vi "LVClass_SlopesPostProcessList AddProcessorTab.vi"(0 "SlopesPostProcessorList in":refnum<class "SlopesPostProcessorList.lvclass">, 5 "Processor List":T1[](array[typedef]), 11 "error in (no error)":errorcluster) -> (4 "SlopesPostProcessorList out":refnum<class "SlopesPostProcessorList.lvclass">, 15 "error out":errorcluster)   [LabVIEW 2020, in "SlopesPostProcessorList.lvclass"]
uses:
  SlopesPostProcessorList.lvclass
  SlopesPostProcessorList - ONE.ctl
  SlopesPostProcessorList - Filter.ctl
  SlopesPostProcessorList - Add lens.ctl
  SlopesPostProcessorList - Double passage.ctl
  HasoSlopes.lvclass
  SlopesPostProcessorList.lvclass/SlopesPostProcessorList.ctl
  Pupil.lvclass
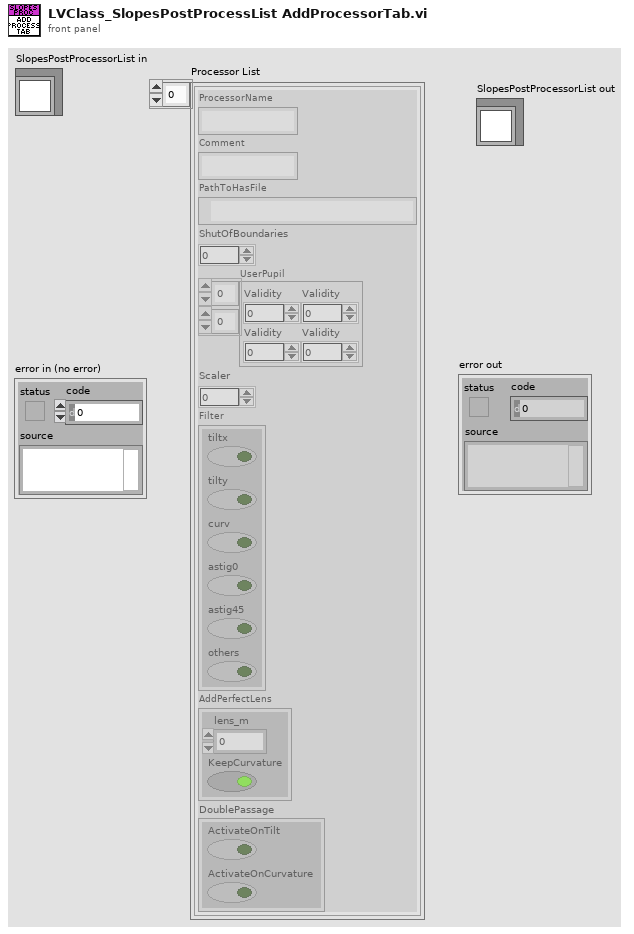
[diagram p1: front panel]
types:
  T1 = typedef "SlopesPostProcessorList - ONE.ctl" = cluster{"ProcessorName":string, "Comment":string, "PathToHasFile":path, "ShutOfBoundaries":u16, "UserPupil":i8[][], "Scaler":sgl, "Filter":T2, "AddPerfectLens":T3, "DoublePassage":T4}
  T2 = typedef "SlopesPostProcessorList - Filter.ctl" = cluster{"tiltx":bool, "tilty":bool, "curv":bool, "astig0":bool, "astig45":bool, "others":bool}
  T3 = typedef "SlopesPostProcessorList - Add lens.ctl" = cluster{"lens_m":sgl, "KeepCurvature":bool}
  T4 = typedef "SlopesPostProcessorList - Double passage.ctl" = cluster{"ActivateOnTilt":bool, "ActivateOnCurvature":bool}
  T5 = typedef "General dimensions definition.ctl" = cluster{"Size":T6, "Step":T7}
  T6 = typedef "Point2D.ctl" = cluster{"X":u32, "Y":u32}
  T7 = typedef "Point2Df.ctl" = cluster{"X":sgl, "Y":sgl}
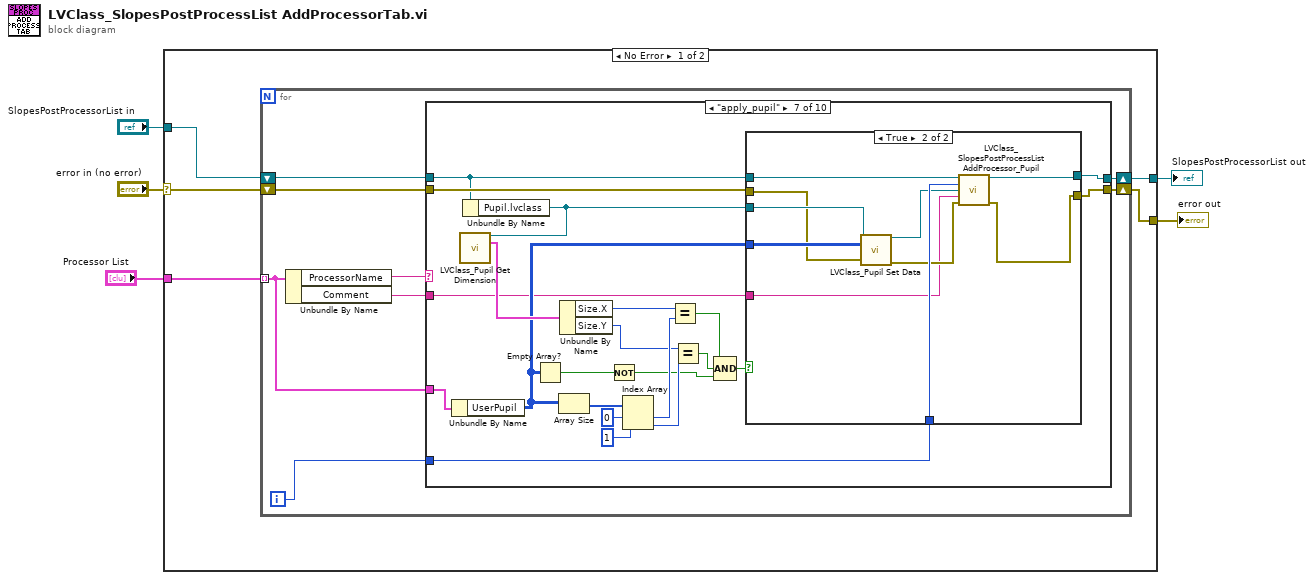
[diagram p0: block diagram]
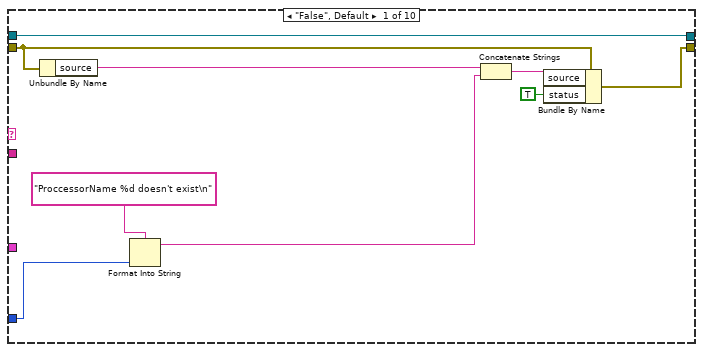
[diagram p2: hidden frame]
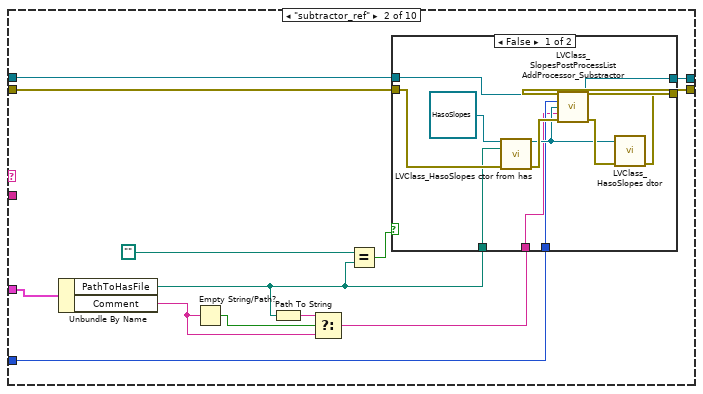
[diagram p3: hidden frame]
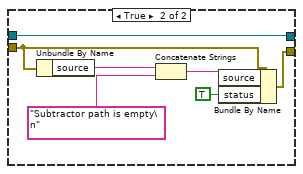
[diagram p4: hidden frame]
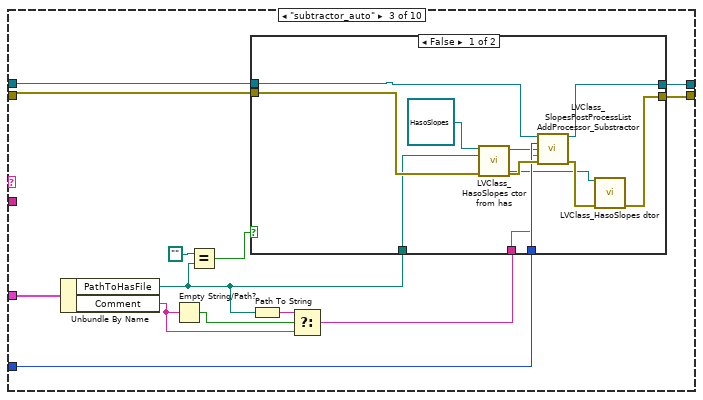
[diagram p5: hidden frame]
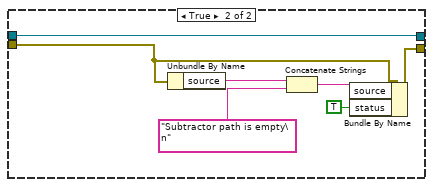
[diagram p6: hidden frame]
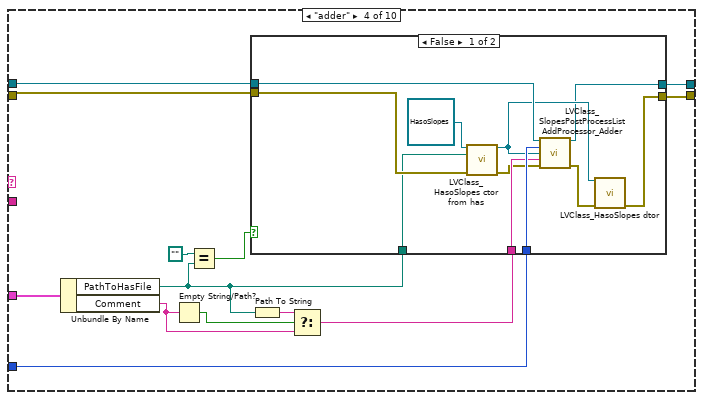
[diagram p7: hidden frame]
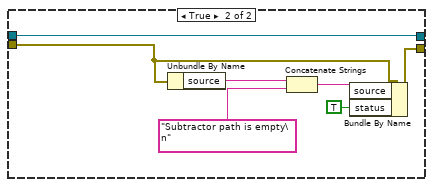
[diagram p8: hidden frame]
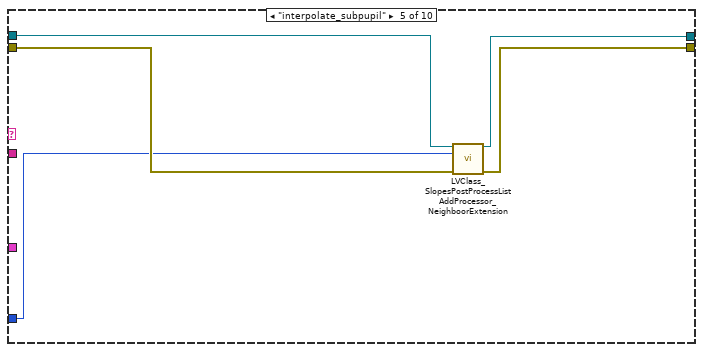
[diagram p9: hidden frame]
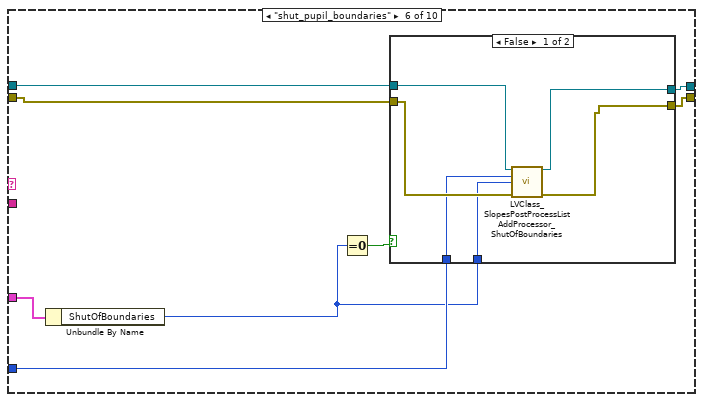
[diagram p10: hidden frame]
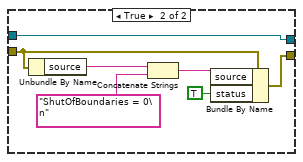
[diagram p11: hidden frame]
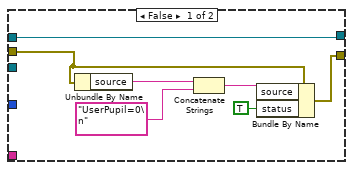
[diagram p12: hidden frame]
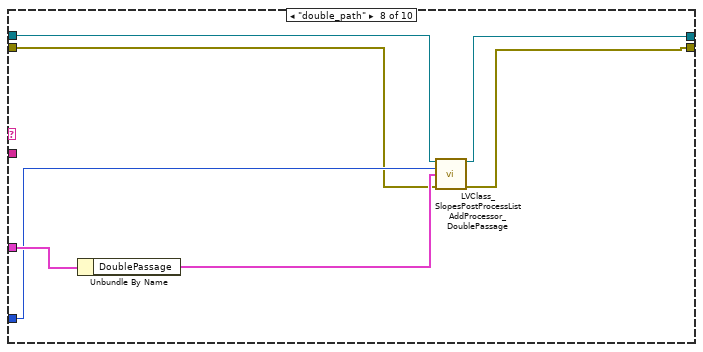
[diagram p13: hidden frame]
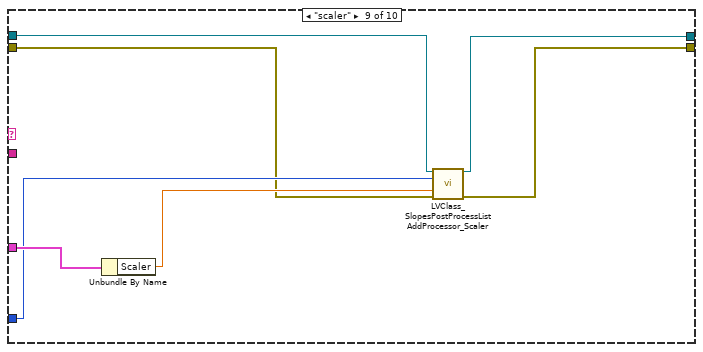
[diagram p14: hidden frame]
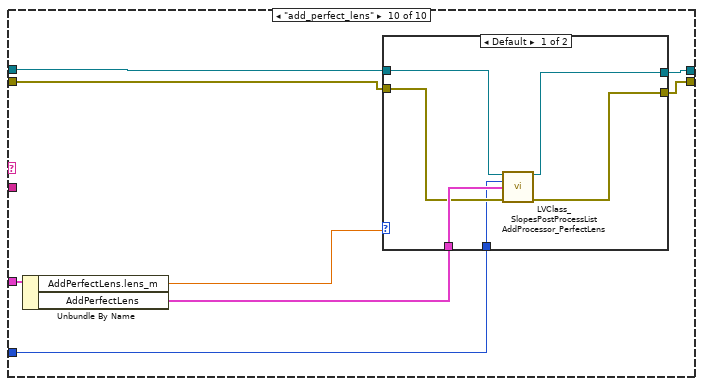
[diagram p15: hidden frame]
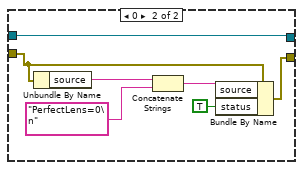
[diagram p16: hidden frame]
diagram:
  n1 = case shown="No Error" "error in (no error)" {
    selector: "error in (no error)" -> [w10 w221]
    tunnel: [w6 w221] -> w4
    tunnel: [w7 w222] -> w2
    tunnel: "SlopesPostProcessorList in" -> [w8 w222]
    tunnel: "Processor List" -> [w9 _]
    frame No Error {
      n2 = for {
        tunnel: w9 -> [w17] mode=indexing
        shift-right: [w15] -> w6
        shift-left: w10 -> [w16]
        shift-right: [w12] -> w7
        shift-left: w8 -> [w13]
        i -> [w14]
        n3 = Unbundle By Name(w17) -> ("ProcessorName"=w18:string, "Comment"=w11:string)
        n4 = case shown="\"apply_pupil\"" w18 {
          tunnel: w17 -> [_ w40 w71 w102 _ w133 w168 w192 w199 w207]
          tunnel: w16 -> [w27 w39 w68 w99 w123 w131 w167 w187 w194 w205]
          tunnel: [w26 w38 w67 w98 w122 w130 w166 w186 w193 w206] -> w15
          tunnel: w14 -> [w22 w33 w64 w95 w121 w127 w163 w190 w196 w200]
          tunnel: w13 -> [w19 w35 w66 w97 w125 w129 w162 w189 w198 w202]
          tunnel: [w19 w34 w65 w96 w124 w128 w164 w188 w197 w201] -> w12
          tunnel: w11 -> [_ _ _ _ _ _ w147 _ _ _]
          frame "False", Default {
            n5 = Unbundle By Name(w27) -> ("source"=w24:string)
            n6 = Format Into String(format string="ProccessorName %d doesn't exist\n" ("source"), w22) -> (resulting string=w21:string)  [unwired: 2 in, 1 out]
            n7 = Concatenate Strings(w24, w21) -> (w23:string)
            n8 = Bundle By Name(cluster=w27, "source"=w23, "status"=TRUE) -> (w26:errorcluster)
          }
          frame "subtractor_ref" {
            n9 = Unbundle By Name(w40) -> ("PathToHasFile"=w29:path, "Comment"=w30:string)
            n10 = Empty String/Path?(string/path=w30) -> (empty?=w31:bool)
            n11 = Path To String(path=w29) -> (string=w32:string)
            n12 = Select(t=w32, s=w31, f=w30) -> (s? t:f=w28:string)
            n13 = Equal?(x=path "", y=w29) -> (x = y?=w36:bool)
            n14 = case shown="False" w36 {
              tunnel: w39 -> [w47 w54]
              tunnel: [w46 w55] -> w38
              tunnel: w35 -> [w45 w52]
              tunnel: [w44 w52] -> w34
              tunnel: w33 -> [w43 _]
              tunnel: w29 -> [w42 _]
              tunnel: w28 -> [w41 _]
              frame False {
                n15 = call "LVClass_HasoSlopes ctor from has.vi"("HasoSlopes (const)"=refnum<class "HasoSlopes.lvclass"> refnum ("HasoSlopes in"), ".has path"=w42, "error in (no error)"=w47) -> ("HasoSlopes (new)"=w48:refnum<class "HasoSlopes.lvclass">, "error out"=w50:errorcluster)  [unwired: 11 in]
                n16 = call "LVClass_SlopesPostProcessList AddProcessor_Substractor.vi"("SlopesPostProcessorList in"=w45, "Position"=w43, "HasoSlopes.lvclass"=w48, "Comment"=w41, "error in (no error)"=w50) -> ("SlopesPostProcessorList out"=w44:refnum<class "SlopesPostProcessorList.lvclass">, "error out"=w49:errorcluster)  [unwired: 9 in]
                n17 = call "LVClass_HasoSlopes dtor.vi"("HasoSlopes in"=w48, "error in (no error)"=w49) -> ("error out"=w46:errorcluster)  [unwired: 12 in, 1 out]
              }
              frame True {
                n18 = Unbundle By Name(w54) -> ("source"=w57:string)
                n19 = Concatenate Strings(w57, "Subtractor path is empty\n" ("source")) -> (w56:string)
                n20 = Bundle By Name(cluster=w54, "source"=w56, "status"=TRUE) -> (w55:errorcluster)
              }
            }
          }
          frame "subtractor_auto" {
            n21 = Unbundle By Name(w71) -> ("PathToHasFile"=w63:path, "Comment"=w61:string)
            n22 = Empty String/Path?(string/path=w61) -> (empty?=w60:bool)
            n23 = Equal?(x=path "", y=w63) -> (x = y?=w69:bool)
            n24 = Path To String(path=w63) -> (string=w62:string)
            n25 = Select(t=w62, s=w60, f=w61) -> (s? t:f=w59:string)
            n26 = case shown="False" w69 {
              tunnel: w68 -> [w81 w85]
              tunnel: [w75 w84] -> w67
              tunnel: w63 -> [w73 _]
              tunnel: w66 -> [w79 w83]
              tunnel: [w78 w83] -> w65
              tunnel: w64 -> [w77 _]
              tunnel: w59 -> [w72 _]
              frame False {
                n27 = call "LVClass_HasoSlopes ctor from has.vi"("HasoSlopes (const)"=refnum<class "HasoSlopes.lvclass"> refnum ("HasoSlopes in"), ".has path"=w73, "error in (no error)"=w81) -> ("HasoSlopes (new)"=w74:refnum<class "HasoSlopes.lvclass">, "error out"=w80:errorcluster)  [unwired: 11 in]
                n28 = call "LVClass_SlopesPostProcessList AddProcessor_Substractor.vi"("SlopesPostProcessorList in"=w79, "Position"=w77, "HasoSlopes.lvclass"=w74, "Comment"=w72, "error in (no error)"=w80) -> ("SlopesPostProcessorList out"=w78:refnum<class "SlopesPostProcessorList.lvclass">, "error out"=w76:errorcluster)  [unwired: 9 in]
                n29 = call "LVClass_HasoSlopes dtor.vi"("HasoSlopes in"=w74, "error in (no error)"=w76) -> ("error out"=w75:errorcluster)  [unwired: 12 in, 1 out]
              }
              frame True {
                n30 = Unbundle By Name(w85) -> ("source"=w88:string)
                n31 = Concatenate Strings(w88, "Subtractor path is empty\n" ("source")) -> (w87:string)
                n32 = Bundle By Name(cluster=w85, "source"=w87, "status"=TRUE) -> (w84:errorcluster)
              }
            }
          }
          frame "adder" {
            n33 = Unbundle By Name(w102) -> ("PathToHasFile"=w94:path, "Comment"=w92:string)
            n34 = Empty String/Path?(string/path=w92) -> (empty?=w91:bool)
            n35 = Equal?(x=path "", y=w94) -> (x = y?=w100:bool)
            n36 = Path To String(path=w94) -> (string=w93:string)
            n37 = Select(t=w93, s=w91, f=w92) -> (s? t:f=w90:string)
            n38 = case shown="False" w100 {
              tunnel: w99 -> [w112 w116]
              tunnel: [w111 w115] -> w98
              tunnel: w94 -> [w110 _]
              tunnel: w97 -> [w109 w114]
              tunnel: [w104 w114] -> w96
              tunnel: w95 -> [w108 _]
              tunnel: w90 -> [w106 _]
              frame False {
                n39 = call "LVClass_HasoSlopes ctor from has.vi"("HasoSlopes (const)"=refnum<class "HasoSlopes.lvclass"> refnum ("HasoSlopes in"), ".has path"=w110, "error in (no error)"=w112) -> ("HasoSlopes (new)"=w107:refnum<class "HasoSlopes.lvclass">, "error out"=w105:errorcluster)  [unwired: 11 in]
                n40 = call "LVClass_SlopesPostProcessList AddProcessor_Adder.vi"("SlopesPostProcessorList in"=w109, "Position"=w108, "HasoSlopes.lvclass"=w107, "Comment"=w106, "error in (no error)"=w105) -> ("SlopesPostProcessorList out"=w104:refnum<class "SlopesPostProcessorList.lvclass">, "error out"=w103:errorcluster)  [unwired: 9 in]
                n41 = call "LVClass_HasoSlopes dtor.vi"("HasoSlopes in"=w107, "error in (no error)"=w103) -> ("error out"=w111:errorcluster)  [unwired: 12 in, 1 out]
              }
              frame True {
                n42 = Unbundle By Name(w116) -> ("source"=w119:string)
                n43 = Concatenate Strings(w119, "Subtractor path is empty\n" ("source")) -> (w118:string)
                n44 = Bundle By Name(cluster=w116, "source"=w118, "status"=TRUE) -> (w115:errorcluster)
              }
            }
          }
          frame "interpolate_subpupil" {
            n45 = call "LVClass_SlopesPostProcessList AddProcessor_NeighboorExtension.vi"("SlopesPostProcessorList in"=w125, "Position"=w121, "error in (no error)"=w123) -> ("SlopesPostProcessorList out"=w124:refnum<class "SlopesPostProcessorList.lvclass">, "error out"=w122:errorcluster)  [unwired: 11 in]
          }
          frame "shut_pupil_boundaries" {
            n46 = Unbundle By Name(w133) -> ("ShutOfBoundaries"=w126:u16)
            n47 = Equal To 0?(x=w126) -> (x = 0?=w132:bool)
            n48 = case shown="False" w132 {
              tunnel: w131 -> [w138 w141]
              tunnel: [w137 w142] -> w130
              tunnel: w129 -> [w139 w140]
              tunnel: [w136 w140] -> w128
              tunnel: w127 -> [w135 _]
              tunnel: w126 -> [w134 _]
              frame False {
                n49 = call "LVClass_SlopesPostProcessList AddProcessor_ShutOfBoundaries.vi"("SlopesPostProcessorList in"=w139, "Position"=w135, "ShutOfBoundaries"=w134, "error in (no error)"=w138) -> ("SlopesPostProcessorList out"=w136:refnum<class "SlopesPostProcessorList.lvclass">, "error out"=w137:errorcluster)  [unwired: 10 in]
              }
              frame True {
                n50 = Unbundle By Name(w141) -> ("source"=w145:string)
                n51 = Concatenate Strings(w145, "ShutOfBoundaries = 0\n" ("source")) -> (w144:string)
                n52 = Bundle By Name(cluster=w141, "source"=w144, "status"=TRUE) -> (w142:errorcluster)
              }
            }
          }
          frame "apply_pupil" {
            n53 = Unbundle By Name(w168) -> ("UserPupil"=w159:i8[][])
            n54 = Unbundle By Name(w162) -> ("Pupil.lvclass"=w161:refnum<class "Pupil.lvclass">)
            n55 = call "LVClass_Pupil Get Dimension.vi"("Pupil in"=w161) -> ("Dimension"=w160:T5)  [unwired: 12 in, 2 out]
            n56 = Empty Array?(array=w159) -> (empty?=w165:bool)
            n57 = Array Size(array=w159) -> (size(s)=w158:i32[])
            n58 = Unbundle By Name(w160) -> ("Size.X"=w155:u32, "Size.Y"=w153:u32)
            n59 = Not(x=w165) -> (.not. x?=w149:bool)
            n60 = Index Array(array=w158, index #1=0 ("index"), index #2=1 ("index")) -> (element #1=w154:i32, element #2=w152:i32)
            n61 = Equal?(x=w155, y=w154) -> (x = y?=w151:bool)
            n62 = Equal?(x=w153, y=w152) -> (x = y?=w150:bool)
            n63 = Compound Arithmetic op=AND(w151, w150, w149) -> (w148:bool)
            n64 = case shown="True" w148 {
              tunnel: w167 -> [w172 w178]
              tunnel: [w171 w177] -> w166
              tunnel: w162 -> [w169 w185]
              tunnel: [w169 w180] -> w164
              tunnel: w163 -> [_ w183]
              tunnel: w159 -> [_ w184]
              tunnel: w161 -> [_ w179]
              tunnel: w147 -> [_ w176]
              frame False {
                n65 = Unbundle By Name(w172) -> ("source"=w174:string)
                n66 = Concatenate Strings(w174, "UserPupil=0\n" ("source")) -> (w173:string)
                n67 = Bundle By Name(cluster=w172, "source"=w173, "status"=TRUE) -> (w171:errorcluster)
              }
              frame True {
                n68 = call "LVClass_Pupil Set Data.vi"("Pupil in"=w179, "Data"=w184, "error in (no error)"=w178) -> ("Pupil out"=w181:refnum<class "Pupil.lvclass">, "error out"=w182:errorcluster)  [unwired: 11 in]
                n69 = call "LVClass_SlopesPostProcessList AddProcessor_Pupil.vi"("SlopesPostProcessorList in"=w185, "Position"=w183, "Pupil.lvclass"=w181, "Comment"=w176, "error in (no error)"=w182) -> ("SlopesPostProcessorList out"=w180:refnum<class "SlopesPostProcessorList.lvclass">, "error out"=w177:errorcluster)  [unwired: 9 in]
              }
            }
          }
          frame "double_path" {
            n70 = Unbundle By Name(w192) -> ("DoublePassage"=w191:T4)
            n71 = call "LVClass_SlopesPostProcessList AddProcessor_DoublePassage.vi"("SlopesPostProcessorList in"=w189, "Position"=w190, "doublePath"=w191, "error in (no error)"=w187) -> ("SlopesPostProcessorList out"=w188:refnum<class "SlopesPostProcessorList.lvclass">, "error out"=w186:errorcluster)  [unwired: 10 in]
          }
          frame "scaler" {
            n72 = Unbundle By Name(w199) -> ("Scaler"=w195:sgl)
            n73 = call "LVClass_SlopesPostProcessList AddProcessor_Scaler.vi"("SlopesPostProcessorList in"=w198, "Position"=w196, "scaler"=w195, "error in (no error)"=w194) -> ("SlopesPostProcessorList out"=w197:refnum<class "SlopesPostProcessorList.lvclass">, "error out"=w193:errorcluster)  [unwired: 10 in]
          }
          frame "add_perfect_lens" {
            n74 = Unbundle By Name(w207) -> ("AddPerfectLens.lens_m"=w204:sgl, "AddPerfectLens"=w203:T3)
            n75 = case shown="Default" w204 {
              tunnel: w205 -> [w209 w217]
              tunnel: [w210 w216] -> w206
              tunnel: w203 -> [w213 _]
              tunnel: w202 -> [w212 w214]
              tunnel: [w211 w214] -> w201
              tunnel: w200 -> [w208 _]
              frame Default {
                n76 = call "LVClass_SlopesPostProcessList AddProcessor_PerfectLens.vi"("SlopesPostProcessorList in"=w212, "Position"=w208, "Perfect lens"=w213, "error in (no error)"=w209) -> ("SlopesPostProcessorList out"=w211:refnum<class "SlopesPostProcessorList.lvclass">, "error out"=w210:errorcluster)  [unwired: 10 in]
              }
              frame 0 {
                n77 = Unbundle By Name(w217) -> ("source"=w219:string)
                n78 = Concatenate Strings(w219, "PerfectLens=0\n" ("source")) -> (w218:string)
                n79 = Bundle By Name(cluster=w217, "source"=w218, "status"=TRUE) -> (w216:errorcluster)
              }
            }
          }
        }
      }
    }
    frame Error {
    }
  }
  "error out" <- w4
  "SlopesPostProcessorList out" <- w2
